vi "SetSourceData.vi"(8 "error in (no error)":errorcluster, 10 "SourceData":dbl, 11 "ChildSource in":refnum<class "ChildSource.lvclass">) -> (0 "error out":errorcluster, 3 "ChildSource out":refnum<class "ChildSource.lvclass">)   [LabVIEW 2023, in "ChildSource.lvclass"]
uses:
  ChildSource.lvclass
  ChildSource.lvclass/ChildSource.ctl
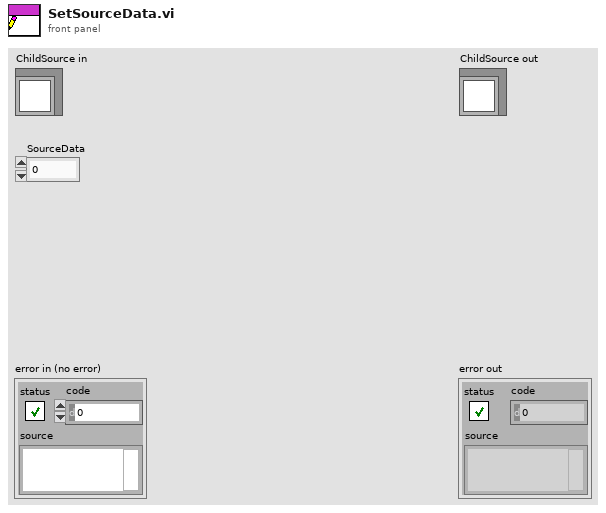
[diagram p1: front panel]
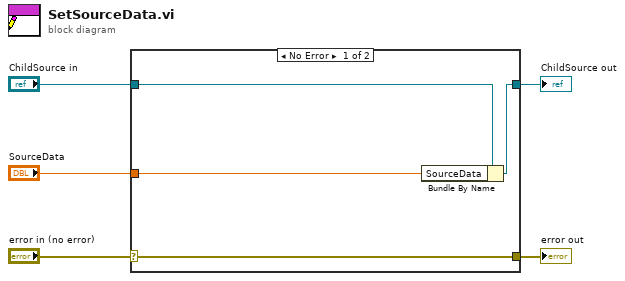
[diagram p0: block diagram]
diagram:
  n1 = case shown="No Error" "error in (no error)" {
    selector: "error in (no error)" -> [w9 w10]
    tunnel: [w9 w10] -> w4
    tunnel: [w7 w11] -> w2
    tunnel: "ChildSource in" -> [w8 w11]
    tunnel: "SourceData" -> [w6 _]
    frame No Error {
      n2 = Bundle By Name(cluster=w8, "SourceData"=w6) -> (w7:refnum<class "ChildSource.lvclass">)
    }
    frame Error {
    }
  }
  "error out" <- w4
  "ChildSource out" <- w2
